vi "Loss测量.vi"(7 "VISA resource name":refnum<visa-resource-name>, 8 "error in (no error)":errorcluster, 10 "Freq":dbl[](array[numeric]), 11 "keysight in":refnum<class "keysight.lvclass">) -> (0 "error out":errorcluster, 1 "S12":dbl[](array[numeric]), 2 "S11":dbl[](array[numeric]), 3 "keysight out":refnum<class "keysight.lvclass">, 4 "S22":dbl[](array[numeric]), 5 "freq":dbl[](array[numeric]), 6 "S21":dbl[](array[numeric]))   [LabVIEW 2015, in "keysight.lvclass"]
uses:
  keysight.lvclass
  E5071C/Agilent ENA Series/Agilent ENA Series.lvlib
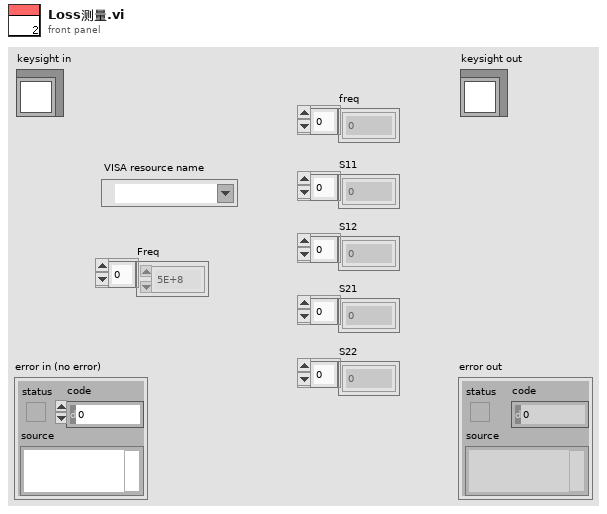
[diagram p1: front panel]
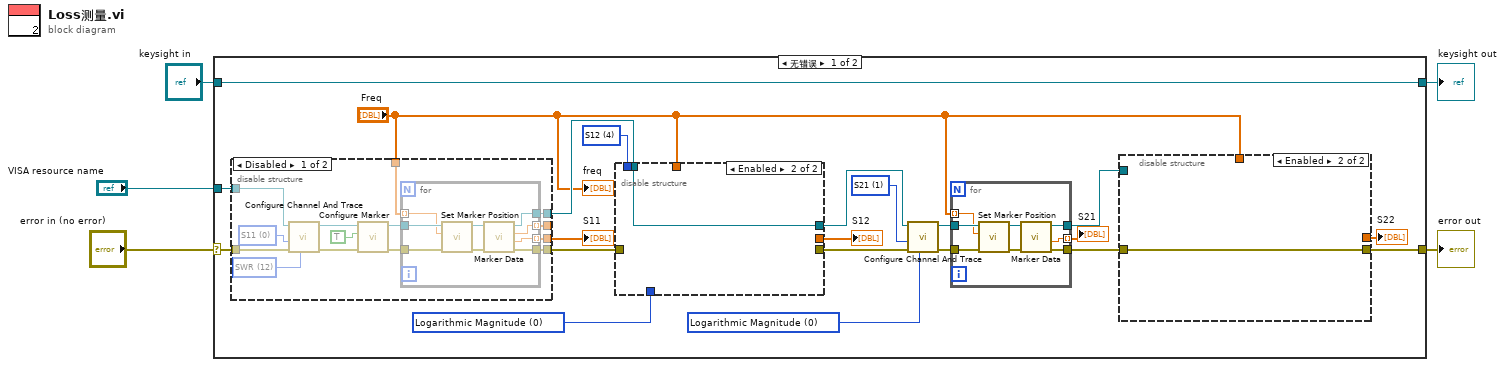
[diagram p0: block diagram]
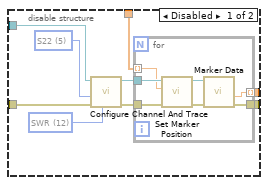
[diagram p2: hidden frame]
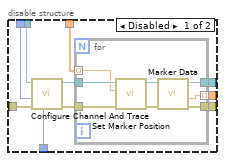
[diagram p3: hidden frame]
diagram:
  n1 = case shown="无错误" "error in (no error)" {
    selector: "error in (no error)" -> [w14 w96]
    tunnel: [w13 w96] -> w1
    tunnel: "VISA resource name" -> [w8 _]
    tunnel: "keysight in" -> [w7 w95]
    tunnel: [w7 w95] -> w3
    frame No Error {
      w21 = u16 0 items=["Logarithmic Magnitude", "Phase", "Group Delay", "Smith Chart  Linear (Lin/Phase)", "Smith Chart  Logarithmic (Log/Phase)", "Smith Chart  Complex (Real/Imag)", "Smith Chart  Impedance (R+jX)", "Smith Chart  Admittance (G+jB)", "Polar Format (Linear)", "Polar Format (Logarithmic)", "Polar Format (Re/Im)", "Linear Magnitude", "SWR", "Real", "Imaginary", "Epanded Phase", "Positive Phase"] ("Data Format (0: Logarithmic Magnitude)")
      w22 = u16 1 items=["S11", "S21", "S31", "S41", "S12", "S22", "S32", "S42", "S13", "S23", "S33", "S43", "S14", "S24", "S34", "S44", "A", "B", "C", "D", "R1", "R2", "R3", "R4", "AUX1", "AUX2", "TR", "T", "R"] ("Measurement Parameters (0: S11)")
      w16 = u16 0 items=["Logarithmic Magnitude", "Phase", "Group Delay", "Smith Chart  Linear (Lin/Phase)", "Smith Chart  Logarithmic (Log/Phase)", "Smith Chart  Complex (Real/Imag)", "Smith Chart  Impedance (R+jX)", "Smith Chart  Admittance (G+jB)", "Polar Format (Linear)", "Polar Format (Logarithmic)", "Polar Format (Re/Im)", "Linear Magnitude", "SWR", "Real", "Imaginary", "Epanded Phase", "Positive Phase"] ("Data Format (0: Logarithmic Magnitude)")
      w15 = u16 4 items=["S11", "S21", "S31", "S41", "S12", "S22", "S32", "S42", "S13", "S23", "S33", "S43", "S14", "S24", "S34", "S44", "A", "B", "C", "D", "R1", "R2", "R3", "R4", "AUX1", "AUX2", "TR", "T", "R"] ("Measurement Parameters (0: S11)")
      n2 = disable-structure shown="Disabled" {
        disable-tunnel: [w76 _] -> w18
        disable-tunnel: [w75 w86] -> w17
        disable-tunnel: w14 -> [w67 _]
        disable-tunnel: [w66 _] -> _
        disable-tunnel: [w65 _] -> w12
        disable-tunnel: w8 -> [w64 w86]
        disable-tunnel: "Freq" -> [w63 _]
        frame Disabled {
          w69 = u16 12 items=["Logarithmic Magnitude", "Phase", "Group Delay", "Smith Chart  Linear (Lin/Phase)", "Smith Chart  Logarithmic (Log/Phase)", "Smith Chart  Complex (Real/Imag)", "Smith Chart  Impedance (R+jX)", "Smith Chart  Admittance (G+jB)", "Polar Format (Linear)", "Polar Format (Logarithmic)", "Polar Format (Re/Im)", "Linear Magnitude", "SWR", "Real", "Imaginary", "Epanded Phase", "Positive Phase"] ("Data Format (0: Logarithmic Magnitude)")
          w68 = u16 0 items=["S11", "S21", "S31", "S41", "S12", "S22", "S32", "S42", "S13", "S23", "S33", "S43", "S14", "S24", "S34", "S44", "A", "B", "C", "D", "R1", "R2", "R3", "R4", "AUX1", "AUX2", "TR", "T", "R"] ("Measurement Parameters (0: S11)")
          n3 = call "Configure Channel And Trace.vi"("Data Format (0: Logarithmic Magnitude)"=w69, "error in (no error)"=w67, "Measurement Parameters (0: S11)"=w68, "VISA resource name"=w64) -> ("error out"=w71:errorcluster, "VISA resource name out"=w70:refnum<visa-resource-name>)  [unwired: 6 in]
          n4 = call "Configure Marker.vi"("error in (no error)"=w71, "Marker State (F: Disabled)"=TRUE, "VISA resource name"=w70) -> ("error out"=w74:errorcluster, "VISA resource name out"=w73:refnum<visa-resource-name>)  [unwired: 7 in]
          n5 = for {
            tunnel: w73 -> [w85]
            tunnel: w74 -> [w84]
            tunnel: [w81] -> w75
            tunnel: [w80] -> w76
            tunnel: [w79] -> w66 mode=indexing
            tunnel: [w78] -> w65 mode=indexing
            tunnel: w63 -> [w77] mode=indexing
            n6 = call "Set Marker Position.vi"("error in (no error)"=w84, "X Value (0.0)"=w77, "VISA resource name"=w85) -> ("error out"=w82:errorcluster, "VISA resource name out"=w83:refnum<visa-resource-name>)  [unwired: 7 in]
            n7 = call "Marker Data.vi"("error in (no error)"=w82, "VISA resource name"=w83) -> ("error out"=w80:errorcluster, "Y Real Value"=w78:dbl, "X Value"=w79:dbl, "VISA resource name out"=w81:refnum<visa-resource-name>)  [unwired: 5 in, 1 out]
          }
        }
        frame Enabled {
        }
      }
      "S11" <- w12
      n8 = disable-structure shown="Enabled" {
        disable-tunnel: [w53 _] -> w24
        disable-tunnel: [w52 w62] -> w23
        disable-tunnel: w18 -> [w49 _]
        disable-tunnel: w17 -> [w48 w62]
        disable-tunnel: w16 -> [w47 _]
        disable-tunnel: w15 -> [w46 _]
        disable-tunnel: [w45 _] -> w11
        disable-tunnel: "Freq" -> [w44 _]
        frame Disabled {
          n9 = call "Configure Channel And Trace.vi"("Data Format (0: Logarithmic Magnitude)"=w47, "error in (no error)"=w49, "Measurement Parameters (0: S11)"=w46, "VISA resource name"=w48) -> ("error out"=w51:errorcluster, "VISA resource name out"=w50:refnum<visa-resource-name>)  [unwired: 6 in]
          n10 = for {
            tunnel: w50 -> [w61]
            tunnel: w51 -> [w60]
            tunnel: [w57] -> w52
            tunnel: [w56] -> w53
            tunnel: [w55] -> w45 mode=indexing
            tunnel: w44 -> [w54] mode=indexing
            n11 = call "Set Marker Position.vi"("error in (no error)"=w60, "X Value (0.0)"=w54, "VISA resource name"=w61) -> ("error out"=w58:errorcluster, "VISA resource name out"=w59:refnum<visa-resource-name>)  [unwired: 7 in]
            n12 = call "Marker Data.vi"("error in (no error)"=w58, "VISA resource name"=w59) -> ("error out"=w56:errorcluster, "Y Real Value"=w55:dbl, "VISA resource name out"=w57:refnum<visa-resource-name>)  [unwired: 5 in, 2 out]
          }
        }
        frame Enabled {
        }
      }
      "S12" <- w11
      n13 = call "Configure Channel And Trace.vi"("Data Format (0: Logarithmic Magnitude)"=w21, "error in (no error)"=w24, "Measurement Parameters (0: S11)"=w22, "VISA resource name"=w23) -> ("error out"=w19:errorcluster, "VISA resource name out"=w20:refnum<visa-resource-name>)  [unwired: 6 in]
      n14 = for {
        tunnel: w20 -> [w94]
        tunnel: w19 -> [w93]
        tunnel: [w90] -> w25
        tunnel: [w89] -> w26
        tunnel: [w88] -> w10 mode=indexing
        tunnel: "Freq" -> [w87] mode=indexing
        n15 = call "Set Marker Position.vi"("error in (no error)"=w93, "X Value (0.0)"=w87, "VISA resource name"=w94) -> ("error out"=w91:errorcluster, "VISA resource name out"=w92:refnum<visa-resource-name>)  [unwired: 7 in]
        n16 = call "Marker Data.vi"("error in (no error)"=w91, "VISA resource name"=w92) -> ("error out"=w89:errorcluster, "Y Real Value"=w88:dbl, "VISA resource name out"=w90:refnum<visa-resource-name>)  [unwired: 5 in, 2 out]
      }
      "S21" <- w10
      n17 = disable-structure shown="Enabled" {
        disable-tunnel: w26 -> [w34 w43]
        disable-tunnel: w25 -> [w33 _]
        disable-tunnel: [w29 w43] -> w13
        disable-tunnel: [w28 _] -> w9
        disable-tunnel: "Freq" -> [w27 _]
        frame Disabled {
          w35 = u16 12 items=["Logarithmic Magnitude", "Phase", "Group Delay", "Smith Chart  Linear (Lin/Phase)", "Smith Chart  Logarithmic (Log/Phase)", "Smith Chart  Complex (Real/Imag)", "Smith Chart  Impedance (R+jX)", "Smith Chart  Admittance (G+jB)", "Polar Format (Linear)", "Polar Format (Logarithmic)", "Polar Format (Re/Im)", "Linear Magnitude", "SWR", "Real", "Imaginary", "Epanded Phase", "Positive Phase"] ("Data Format (0: Logarithmic Magnitude)")
          w30 = u16 5 items=["S11", "S21", "S31", "S41", "S12", "S22", "S32", "S42", "S13", "S23", "S33", "S43", "S14", "S24", "S34", "S44", "A", "B", "C", "D", "R1", "R2", "R3", "R4", "AUX1", "AUX2", "TR", "T", "R"] ("Measurement Parameters (0: S11)")
          n18 = call "Configure Channel And Trace.vi"("Data Format (0: Logarithmic Magnitude)"=w35, "error in (no error)"=w34, "Measurement Parameters (0: S11)"=w30, "VISA resource name"=w33) -> ("error out"=w32:errorcluster, "VISA resource name out"=w31:refnum<visa-resource-name>)  [unwired: 6 in]
          n19 = for {
            tunnel: w31 -> [w42]
            tunnel: w32 -> [w41]
            tunnel: [w38] -> w29
            tunnel: [w37] -> w28 mode=indexing
            tunnel: w27 -> [w36] mode=indexing
            n20 = call "Set Marker Position.vi"("error in (no error)"=w41, "X Value (0.0)"=w36, "VISA resource name"=w42) -> ("error out"=w39:errorcluster, "VISA resource name out"=w40:refnum<visa-resource-name>)  [unwired: 7 in]
            n21 = call "Marker Data.vi"("error in (no error)"=w39, "VISA resource name"=w40) -> ("error out"=w38:errorcluster, "Y Real Value"=w37:dbl)  [unwired: 5 in, 3 out]
          }
        }
        frame Enabled {
        }
      }
      "S22" <- w9
      "freq" <- "Freq"
    }
    frame Error {
    }
  }
  "error out" <- w1
  "keysight out" <- w3
